vi "Set Delay.vi"(8 "error in (no error)":errorcluster, 10 "delay (0)":i32, 11 "VISA resource name":refnum<visa-resource-name>) -> (0 "error out":errorcluster, 3 "VISA resource name out":refnum<visa-resource-name>)   [LabVIEW 2024, in "Detector SCPI.lvlib"]
doc: "Set delay between readings for oversampled and burst modes"
uses:
  <instrlib>/Detector SCPI/Detector SCPI.lvlib
panel:
  out "Error Message":string
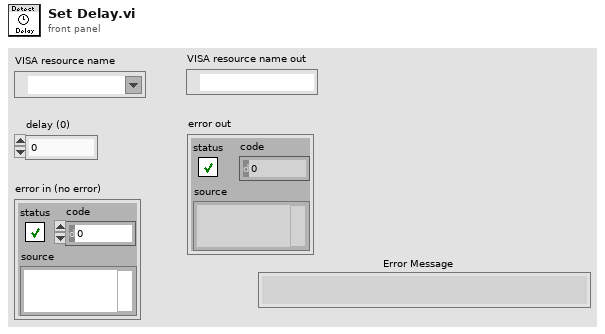
[diagram p1: front panel]
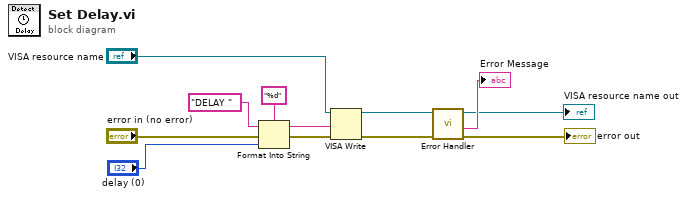
[diagram p0: block diagram]
diagram:
  n1 = Format Into String(format string="%d", initial string="DELAY " ("command"), error in="error in (no error)", "delay (0)") -> (resulting string=w6:string, error out=w10:errorcluster)
  n2 = VISA Write(VISA resource name="VISA resource name", write buffer=w6, error in (no error)=w10) -> (VISA resource name out=w4:refnum<visa-resource-name>, error out=w3:errorcluster)  [unwired: 1 out]
  n3 = call <instrlib>:"Error Handler.vi"("error in (no error)"=w3, "VISA resource name"=w4) -> ("error out"=→"error out":errorcluster, "Error Message"=→"Error Message":string, "VISA resource name out"=→"VISA resource name out":refnum<visa-resource-name>)  [unwired: 7 in]
